vi "qCTI.vi"(0 "System no.":i32=1 min=1 max=4 step=1, 2 "TriggerIn to query":string[](array[string]), 3 "CTI parameter ID":i32[](array[numeric]), 4 "All Triggers?":bool, 5 "error in":errorcluster) -> (15 "Parameter value":string[](array[string]), 16 "TriggerIn to query out":string[](array[string]), 17 "CTI parameter ID out":i32[](array[numeric]), 19 "error out":errorcluster)   [LabVIEW 2020]
doc: "Returns the Trigger Input configuration for the given trigger input line. See user manual for available TriggerIn IDs and CTI parameter IDs.\n\nE-709:"
uses:
  Communication/Global1.vi
panel:
  # "Returns the Trigger Input configuration for the given trigger input line."
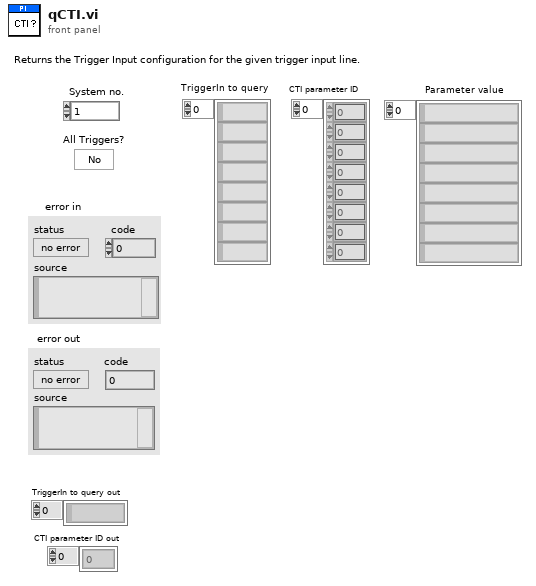
[diagram p1: front panel]
types:
  T1 = typedef "Syntax.ctl" = enum16{"GCS 1.0", "GCS 2.0", "GCS 3.0"}
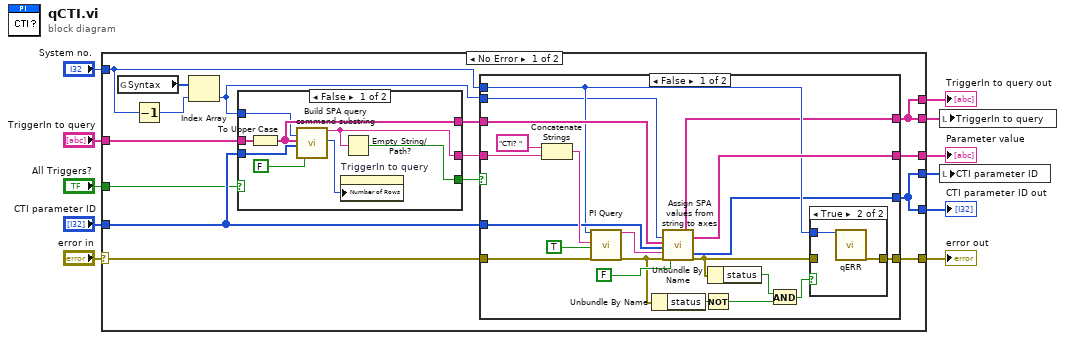
[diagram p0: block diagram]
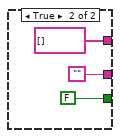
[diagram p2: hidden frame]
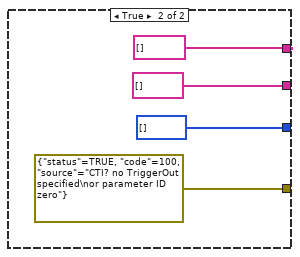
[diagram p4: hidden frame]
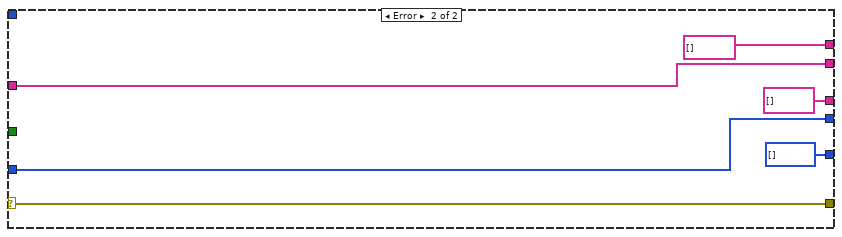
[diagram p5: hidden frame]
diagram:
  n1 = case shown="No Error" "error in" {
    selector: "error in" -> [w15 w70]
    tunnel: "TriggerIn to query" -> [w26 w66]
    tunnel: "System no." -> [w14 _]
    tunnel: "CTI parameter ID" -> [w23 w68]
    tunnel: [w22 w70] -> w8
    tunnel: "All Triggers?" -> [w20 _]
    tunnel: [w19 string[] [] ("Parameter strings")] -> w6
    tunnel: [w12 i32[] [] ("Parameter no. out")] -> w4
    tunnel: [w13 w66] -> w3
    tunnel: [w13 string[] [] ("Queried axes out")] -> w2
    tunnel: [w12 w68] -> w1
    frame No Error {
      n2 = global read "Global1.vi" "Syntax"() -> (w17:T1[])
      n3 = Decrement(x=w14) -> (x-1=w18:i32)
      n4 = Index Array(array=w17, index=w18) -> (element=w16:T1)
      n5 = case shown="False" w20 {
        tunnel: w26 -> [w34 _]
        tunnel: [w28 "" ("Command substring")] -> w25
        tunnel: [w33 string[] [] ("Designator to query")] -> w24
        tunnel: w23 -> [w32 _]
        tunnel: [w27 FALSE] -> w21
        tunnel: w16 -> [w31 _]
        frame False {
          n6 = To Upper Case(1:w34) -> (0:w33:string[])
          n7 = call "Build SPA query command substring.vi"("Syntax"=w31, "Axes to query"=w33, "Parameter number"=w32, "Parameter no. format \n(Decimal: FALSE)"=FALSE ("Parameter no. format \n(Decimal: FALSE)")) -> ("Command substring"=w28:string, "Number of rows"=w30:u32)  [unwired: 3 in, 11 out]
          n8 = property on="TriggerIn to query" class="Arr (strict)"("Number of Rows"=w30) -> ()  [unwired: 2 in, 2 out]
          n9 = Empty String/Path?(string/path=w28) -> (empty?=w27:bool)
        }
        frame True {
        }
      }
      n10 = case shown="False" w21 {
        tunnel: w15 -> [w47 _]
        tunnel: w25 -> [w55 _]
        tunnel: w24 -> [w54 _]
        tunnel: w14 -> [w46 _]
        tunnel: w23 -> [w53 _]
        tunnel: [w49 errorcluster {"status"=TRUE, "code"=100, "source"="CTI? no TriggerOut specified\nor parameter ID zero"} ("error out")] -> w22
        tunnel: [w48 string[] [] ("Parameter strings")] -> w19
        tunnel: w16 -> [w45 _]
        tunnel: [w39 i32[] [] ("Parameter no. out")] -> w12
        tunnel: [w38 string[] [] ("Queried axes out")] -> w13
        frame False {
          n11 = Concatenate Strings("CTI? ", w55) -> (w56:string)
          n12 = call "PI Query.vi"("System no."=w46, "String to send"=w56, "Attach termination char.?"=TRUE ("Attach Linefeed?"), "error in"=w47) -> ("String read"=w41:string, "error out"=w40:errorcluster)  [unwired: 3 in, 11 out]
          n13 = Unbundle By Name(w40) -> ("status"=w42:bool)
          n14 = call "Assign SPA values from string to axes.vi"("Syntax"=w45, "Queried axes"=w54, "Parameter no."=w53, "Input string"=w41, "error in"=w40, "Parameter no. format \n(Decimal: FALSE)"=FALSE ("Parameter no. format \n(Decimal: FALSE)")) -> ("Parameter no. out"=w39:i32[], "Queried axes out"=w38:string[], "Parameter strings"=w48:string[], "error out"=w50:errorcluster)  [unwired: 2 in, 8 out]
          n15 = Not(x=w42) -> (.not. x?=w43:bool)
          n16 = Unbundle By Name(w50) -> ("status"=w52:bool)
          n17 = And(x=w52, y=w43) -> (x .and. y?=w51:bool)
          n18 = case shown="True" w51 {
            tunnel: w50 -> [w59 _]
            tunnel: [w59 w60] -> w49
            tunnel: w46 -> [_ w61]
            frame False {
            }
            frame True {
              n19 = call "qERR.vi"("System no."=w61) -> ("error out"=w60:errorcluster)  [unwired: 1 in, 17 out]
            }
          }
        }
        frame True {
        }
      }
    }
    frame Error {
    }
  }
  "error out" <- w8
  "Parameter value" <- w6
  "CTI parameter ID out" <- w4
  "TriggerIn to query out" <- w2
  n20 = local write "TriggerIn to query"(w3) -> ()
  n21 = local write "CTI parameter ID"(w1) -> ()
